vi "test.vi"() -> ()   [LabVIEW 2022 SP3]
uses:
  Abstract Model/Abstract Model.lvlibp/Abstract Model.lvclass
  <vilib>/Utility/LVLibp/NI_PackedLibraryUtility.lvlib
panel:
  out "changed data":string
  out "value":string
  out "appended path 2":path
  out "appended path":path
  out "path":path
  out "Map 4":map{string, i32}(c390)
  out "Map 3":map{string, i32}(c390)
  out "thread number out":i32
  out "Map 2":map{string, i32}(c390)
  out "Map":map{string, i32}(c390)
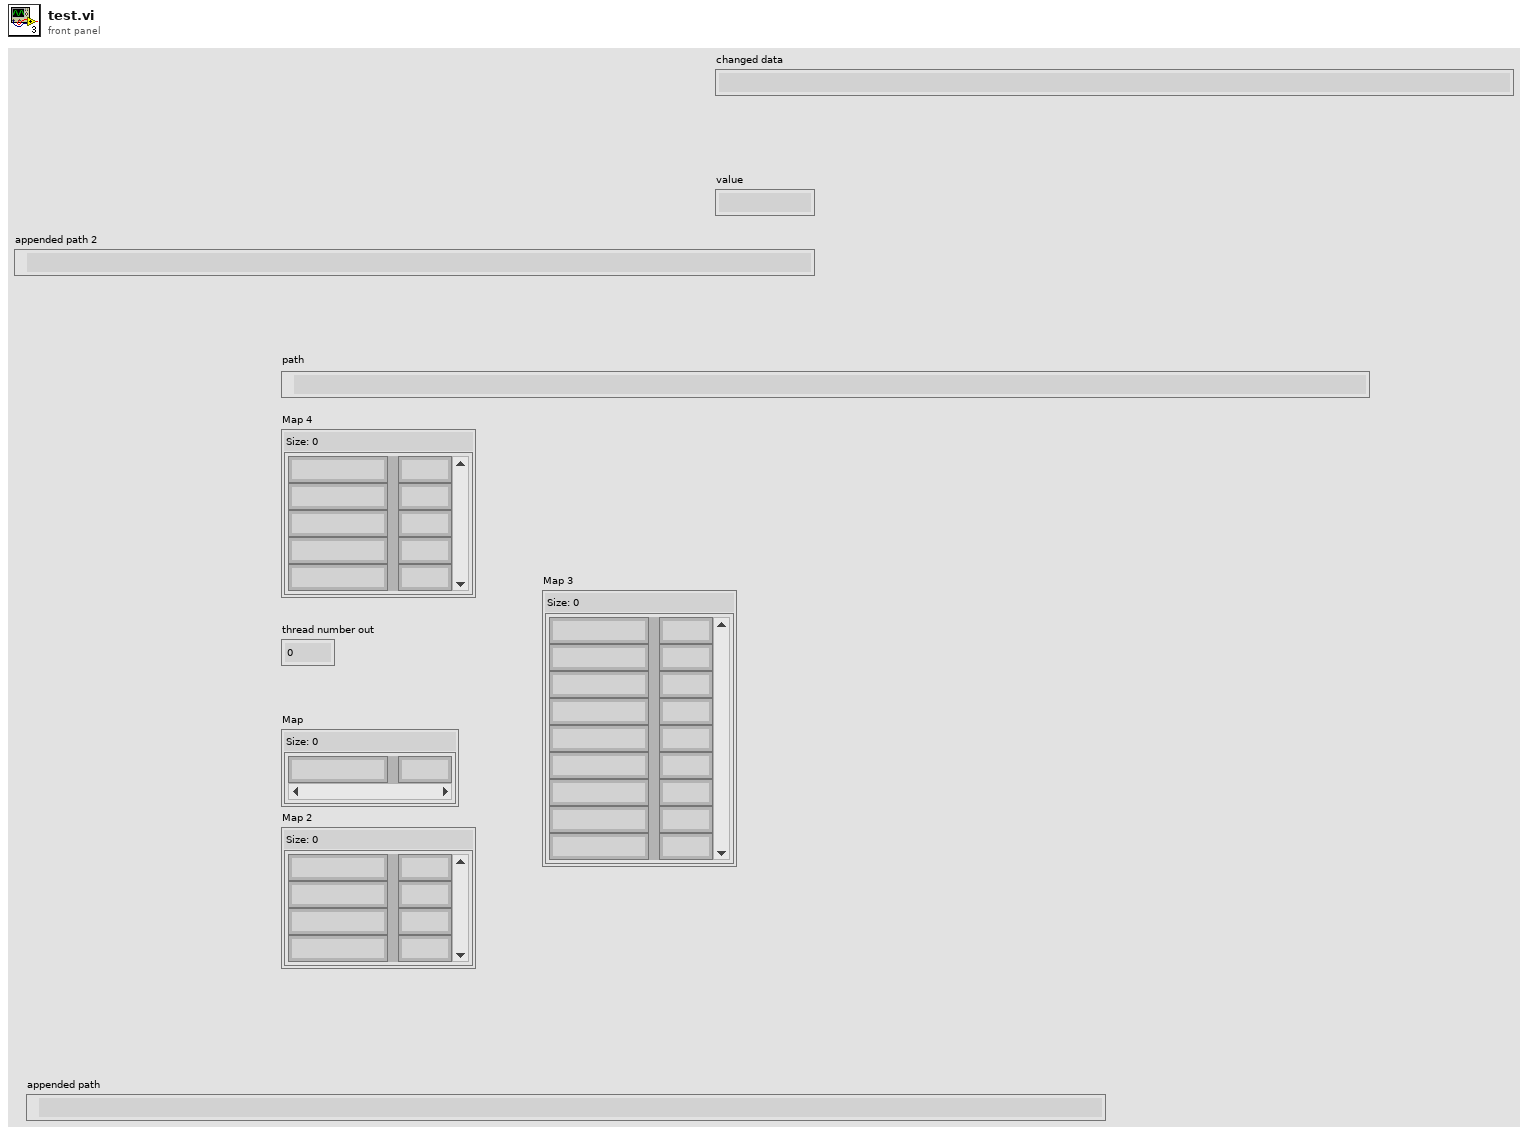
[diagram p1: front panel]
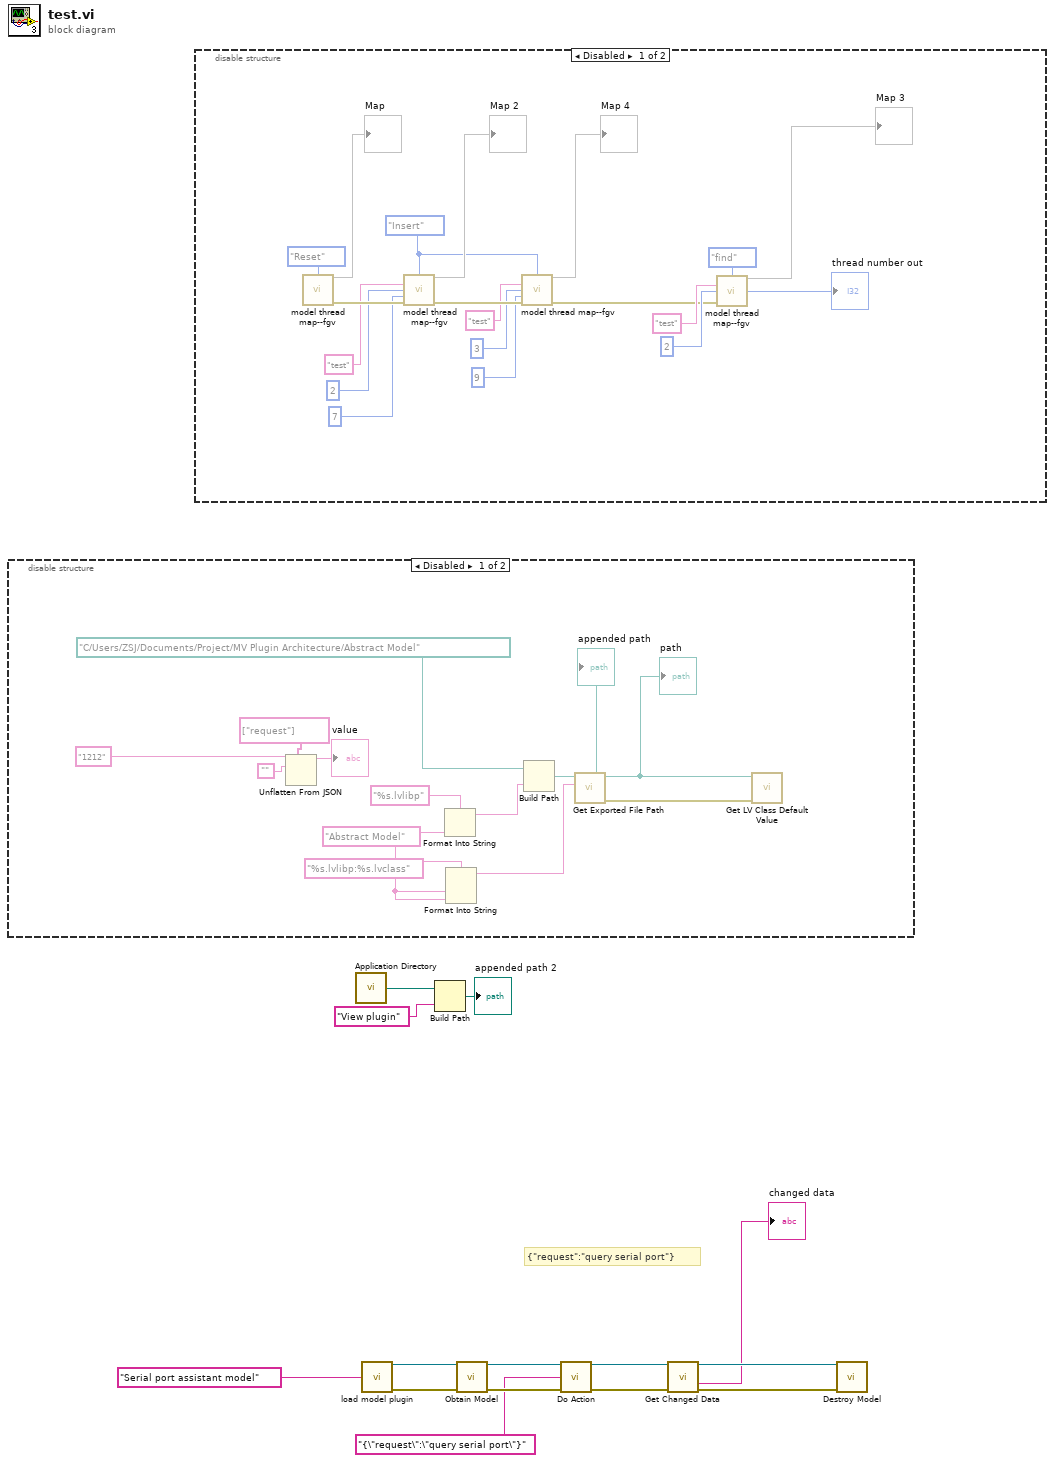
[diagram p0: block diagram]
diagram:
  # "{\"request\":\"query serial port\"}"
  n1 = disable-structure shown="Disabled" {
    frame Disabled {
      w21 = "Abstract Model"
      n2 = Unflatten From JSON(path=string[] ["request"], JSON string="1212", type and defaults="") -> (value=→"value":string)  [unwired: 4 in, 1 out]
      n3 = Format Into String(format string="%s.lvlibp", w21) -> (resulting string=w26:string)  [unwired: 2 in, 1 out]
      n4 = Format Into String(format string="%s.lvlibp:%s.lvclass", w21, w21) -> (resulting string=w23:string)  [unwired: 2 in, 1 out]
      n5 = Build Path(base path=path "C:/Users/ZSJ/Documents/Project/MV Plugin Architecture/Abstract Model" ("Plugins Directory"), name or relative path=w26) -> (appended path=w25:path)
      "appended path" <- w25
      n6 = call <vilib>:"Get Exported File Path.vi"("qualified name"=w23, "packed library path"=w25) -> ("error out"=w20:errorcluster, "path"=w19:path)  [unwired: 8 in]
      "path" <- w19
      n7 = call <vilib>:"Get LV Class Default Value.vi"("error in (no error)"=w20, "class path"=w19) -> ()  [unwired: 8 in, 2 out]
    }
    frame Enabled {
    }
  }
  n8 = disable-structure shown="Disabled" {
    frame Disabled {
      w32 = enum16{"Reset", "Insert", "find"}."Insert" ("operation")
      n9 = call "model thread map--fgv.vi"("operation"=enum16{"Reset", "Insert", "find"}."Reset") -> ("Map"=→"Map":map{string, i32}, "error out"=w45:errorcluster)  [unwired: 10 in, 3 out]
      n10 = call "model thread map--fgv.vi"("operation"=w32, "model name in"="test" ("model name"), "model number in"=2 ("model number"), "thread number In"=7, "error in (no error)"=w45) -> ("Map"=→"Map 2":map{string, i32}, "error out"=w34:errorcluster)  [unwired: 6 in, 3 out]
      n11 = call "model thread map--fgv.vi"("operation"=w32, "model name in"="test", "model number in"=3, "thread number In"=9, "error in (no error)"=w34) -> ("Map"=→"Map 4":map{string, i32}, "error out"=w33:errorcluster)  [unwired: 6 in, 3 out]
      n12 = call "model thread map--fgv.vi"("operation"=enum16{"Reset", "Insert", "find"}."find", "model name in"="test" ("model name"), "model number in"=2 ("model number"), "error in (no error)"=w33) -> ("Map"=→"Map 3":map{string, i32}, "model number out"=→"thread number out":i32)  [unwired: 7 in, 3 out]
    }
    frame Enabled {
    }
  }
  n13 = call <vilib>:"Application Directory.vi"() -> ("Application Directory"=w14:path)
  n14 = call "load model plugin.vi"("model name"="Serial port assistant model") -> ("Model plugin"=w10:refnum<class "Abstract Model.lvclass">, "error out"=w11:errorcluster)  [unwired: 13 in]
  n15 = Build Path(base path=w14, name or relative path="View plugin") -> (appended path=→"appended path 2":path)
  n16 = call-dynamic "Obtain Model.vi"("Abstract Model in"=w10, "error in (no error)"=w11) -> ("Abstract Model out"=w7:refnum<class "Abstract Model.lvclass">, "error out"=w8:errorcluster)  [unwired: 12 in]
  n17 = call-dynamic "Do Action.vi"("Abstract Model in"=w7, "request"="{\"request\":\"query serial port\"}", "error in (no error)"=w8) -> ("Abstract Model out"=w5:refnum<class "Abstract Model.lvclass">, "error out"=w6:errorcluster)  [unwired: 11 in]
  n18 = call-dynamic "Get Changed Data.vi"("Abstract Model in"=w5, "error in (no error)"=w6) -> ("Abstract Model out"=w4:refnum<class "Abstract Model.lvclass">, "changed data"=→"changed data":string, "error out"=w3:errorcluster)  [unwired: 9 in, 2 out]
  n19 = call-dynamic "Destroy Model.vi"("Abstract Model in"=w4, "error in (no error)"=w3) -> ()  [unwired: 12 in, 2 out]
